vi "Configuration Panel.vi"(8 "error in":errorcluster, 11 "Main Data Buffer In":T2) -> (0 "error out":errorcluster, 3 "Main Data Buffer Out":T2)   [LabVIEW 2020, in "SECS Bridge.lvlib"]
uses:
  SECS Bridge.lvlib
  Main Data Buffer.ctl
  SECS Communication/HSMS Class/HSMS Class.lvclass
  SECS Communication/SECS Data Class/SECS Data Class.lvclass
  SECS Scenarios/Scenarios Class/Scenarios Class.lvclass
  Configuration.ctl
  File FGV Method.ctl
  SECS Communication/HSMS Class/HSMS Class.lvclass/HSMS Class.ctl
  SECS Communication/HSMS Class/Write T3(Reply Timeout).vi
  SECS Communication/HSMS Class/Write T5(Separation Timeout).vi
  SECS Communication/HSMS Class/Write T6(Control Timeout).vi
  SECS Communication/HSMS Class/Write T7(Not Selected Timeout).vi
  SECS Communication/HSMS Class/Write T8(Inter-Character Timeout).vi
  SECS Communication/HSMS Class/Write Session ID.vi
  SECS Communication/HSMS Class/Write Log Path.vi
  PPL/Universal Function.lvlibp
panel:
  in  "Reload":bool
  in  "Cancel":bool
  in  "OK":bool
  in  "Configuration":T1={"T3(Reply Timeout)"=45000, "T5(Separation Timeout)"=10000, "T6(Control Timeout)"=5000, "T7(Not Selected Timeout)"=1000, "T8(Inter-Character Timeout)"=5000, "Session ID"=0, "Log Path"=path "D:/SECS", "IP Address"="", "Port"=5000}
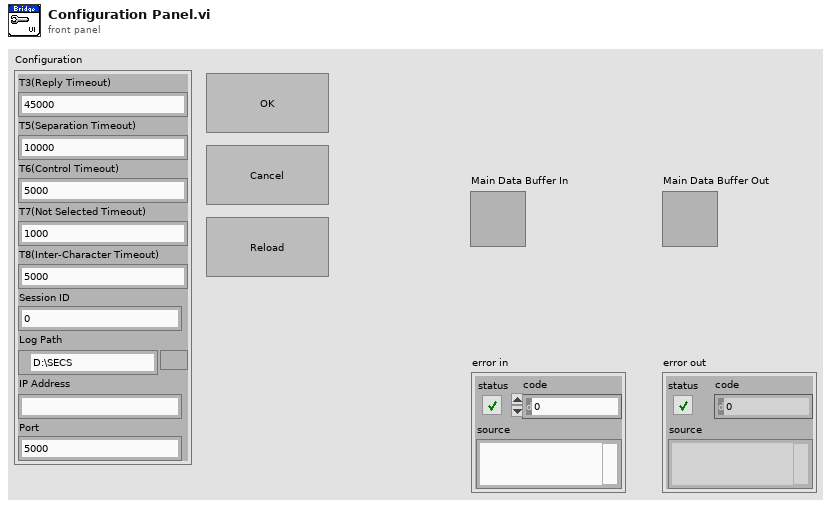
[diagram p1: front panel]
types:
  T1 = typedef "SECS Bridge.lvlib/Configuration.ctl" = cluster{"T3(Reply Timeout)":i32, "T5(Separation Timeout)":i32, "T6(Control Timeout)":i32, "T7(Not Selected Timeout)":i32, "T8(Inter-Character Timeout)":i32, "Session ID":u16, "Log Path":path, "IP Address":string, "Port":u16}
  T2 = typedef "SECS Bridge.lvlib/Main Data Buffer.ctl" = cluster{"HSMS Class":refnum<class "HSMS Class.lvclass">, "SECS Data Class":refnum<class "SECS Data Class.lvclass">, "Scenarios Class":refnum<class "Scenarios Class.lvclass">, "VI Refnum":refnum<vi>, "Ctl Refnum Map":map{string, refnum<vi>}, "Timeout":i32, "Notifier Data":string[], "Event Refnum":refnum<event-registration>}
  T3 = typedef "SECS Bridge.lvlib/File FGV Method.ctl" = enum16{"Get", "Put", "Read", "Write"}
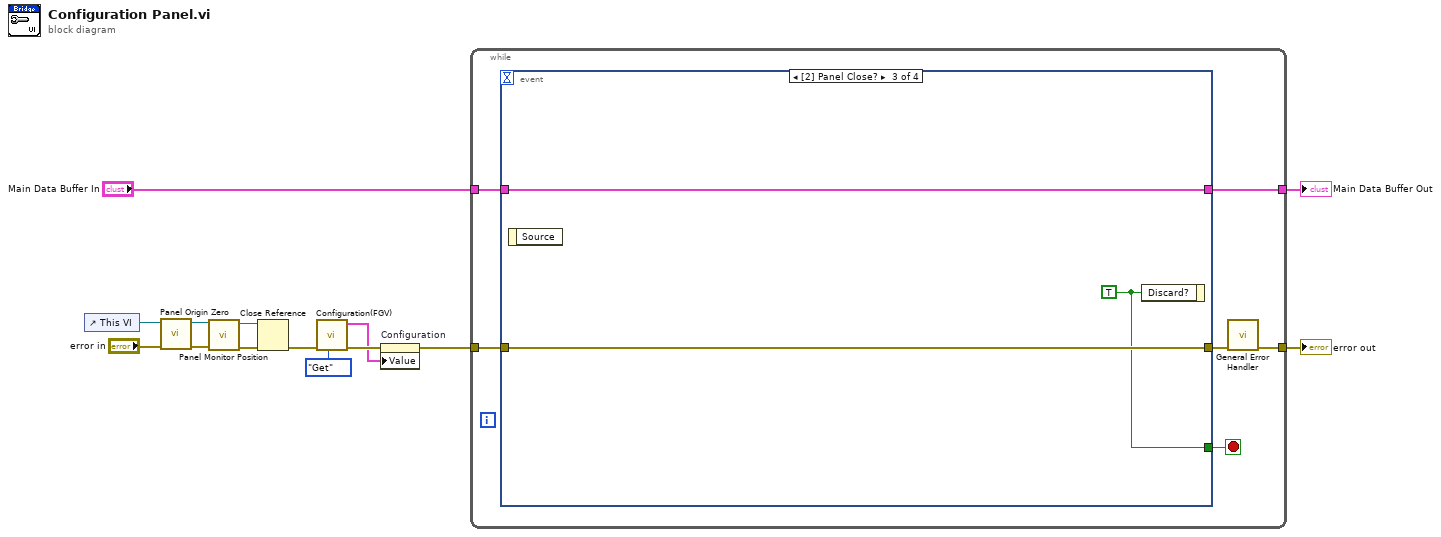
[diagram p0: block diagram]
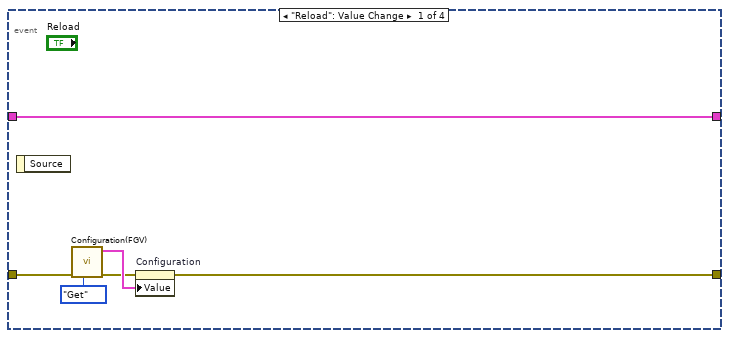
[diagram p2: hidden frame]
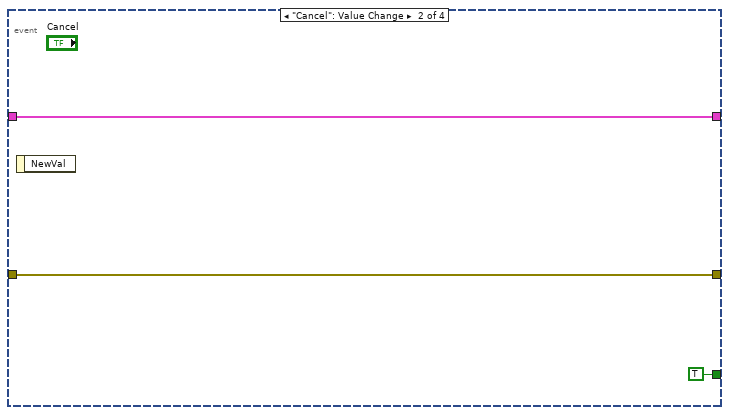
[diagram p3: hidden frame]
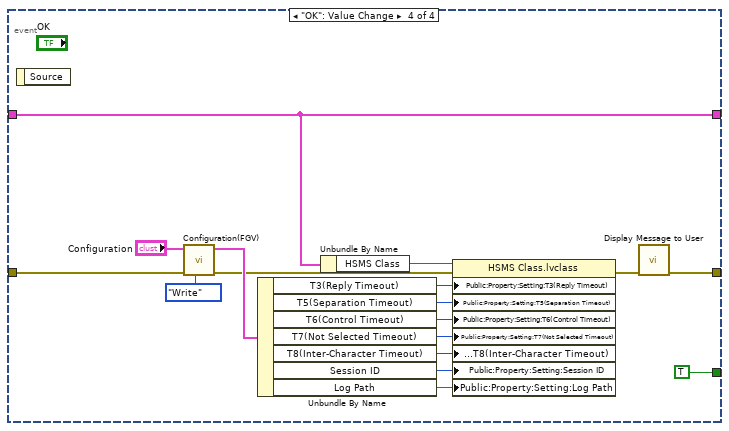
[diagram p4: hidden frame]
diagram:
  n1 = control-ref of="This VI"() -> (w12:refnum<vi>)
  n2 = call "Panel Origin Zero.vi"("error in"="error in", "VI Refnum In"=w12) -> ("error out"=w13:errorcluster, "VI Refnum Out"=w14:refnum<vi>)  [unwired: 8 in]
  n3 = call "Panel Monitor Position.vi"("error in"=w13, "VI Refnum In"=w14) -> ("error out"=w9:errorcluster, "VI Refnum Out"=w10:refnum<vi>)  [unwired: 8 in]
  n4 = Close Reference(reference=w10, error in (no error)=w9) -> (error out=w8:errorcluster)
  n5 = call "Configuration(FGV).vi"("File FGV Method"=File_FGV_Method."Get", "error in"=w8) -> ("error out"=w6:errorcluster, "Configuration Out"=w5:T1)  [unwired: 8 in]
  n6 = property on="Configuration" class="Clust (strict)"(error in=w6, "Value"=w5) -> (error out=w3:errorcluster)  [unwired: 1 in, 1 out]
  n7 = while {
    tunnel: w3 -> [w20]
    tunnel: "Main Data Buffer In" -> [w19]
    tunnel: [w18] -> w1
    tunnel: [w15] -> w2
    stop <- w17 stop-if-true
    n8 = event shown="[2] Panel Close?" {
      selector: _ -> [_ _ _ _]
      dyn-events: _ -> [_ _ _ _]
      timeout: _ -> [_ _ _ _]
      tunnel: w20 -> [w23 w28 w31 w49]
      tunnel: w19 -> [w22 w29 w32 w45]
      tunnel: [w22 w29 w32 w45] -> w18
      tunnel: [w21 w28 w31 w34] -> w16
      tunnel: [_ TRUE w30 TRUE] -> w17
      event "Reload": Value Change {
        n9 = event-data() -> ()  [unwired: 1 in, 1 out]
        n10 = call "Configuration(FGV).vi"("File FGV Method"=File_FGV_Method."Get", "error in"=w23) -> ("error out"=w25:errorcluster, "Configuration Out"=w26:T1)  [unwired: 8 in]
        n11 = property on="Configuration" class="Clust (strict)"(error in=w25, "Value"=w26) -> (error out=w21:errorcluster)  [unwired: 1 in, 1 out]
      }
      event "Cancel": Value Change {
        n12 = event-data() -> ()  [unwired: 1 in, 1 out]
      }
      event Panel Close? {
        w30 = TRUE ("Discard?")
        n13 = event-data() -> ()  [unwired: 1 in, 1 out]
        n14 = event-data("Discard?"=w30) -> ()  [unwired: 1 in, 1 out]
      }
      event "OK": Value Change {
        n15 = event-data() -> ()  [unwired: 1 in, 1 out]
        n16 = call "Configuration(FGV).vi"("File FGV Method"=File_FGV_Method."Write", "error in"=w49, "Configuration In"="Configuration") -> ("error out"=w44:errorcluster, "Configuration Out"=w46:T1)  [unwired: 7 in]
        n17 = Unbundle By Name(w46) -> ("T3(Reply Timeout)"=w42:i32, "T5(Separation Timeout)"=w41:i32, "T6(Control Timeout)"=w40:i32, "T7(Not Selected Timeout)"=w39:i32, "T8(Inter-Character Timeout)"=w38:i32, "Session ID"=w37:u16, "Log Path"=w36:path)
        n18 = Unbundle By Name(w45) -> ("HSMS Class"=w43:refnum<class "HSMS Class.lvclass">)
        n19 = property class="HSMS Class.lvclass"(reference=w43, error in=w44, "Public:Property:Setting:T3(Reply Timeout)"=w42, "Public:Property:Setting:T5(Separation Timeout)"=w41, "Public:Property:Setting:T6(Control Timeout)"=w40, "Public:Property:Setting:T7(Not Selected Timeout)"=w39, "Public:Property:Setting:T8(Inter-Character Timeout)"=w38, "Public:Property:Setting:Session ID"=w37, "Public:Property:Setting:Log Path"=w36) -> (error out=w35:errorcluster)  [unwired: 1 out]
        n20 = call "Display Message to User"("error in (no error)"=w35) -> ("error out"=w34:errorcluster)  [unwired: 9 in, 1 out]
      }
    }
    n21 = call <vilib>:"General Error Handler.vi"("error in (no error)"=w16) -> ("error out"=w15:errorcluster)  [unwired: 10 in, 4 out]
  }
  "error out" <- w2
  "Main Data Buffer Out" <- w1
